vi "FollowerWall.vi"() -> ()   [LabVIEW 2016]
uses:
  <vilib>/NXT/Block Support/NXT_InputPort.ctl
  <vilib>/NXT/Block Support/NXT_TimerIndex.ctl
  <vilib>/NXT/Block Support/NXT_OutputPort.ctl
  <vilib>/NXT/Dual Mode Library/Sensors/EV3_Gyro_Reset.vi
  <vilib>/NXT/Dual Mode Library/Sensors/EV3_Gyro_Angle.vi
  <vilib>/NXT/Dual Mode Library/Sensors/EV3_Gyro_Rate.vi
  <vilib>/NXT/Dual Mode Library/Sensors/Reset_Timer.vi
  <vilib>/NXT/Dual Mode Library/Sensors/EV3_Color_Reflect.vi
  <vilib>/NXT/Dual Mode Library/Sensors/Read_Timer.vi
  <vilib>/NXT/Dual Mode Library/Sensors/EV3_Ultrasonic_CM.vi
  <vilib>/NXT/Dual Mode Library/Display/drawText_Right.vi
  <vilib>/NXT/Dual Mode Library/prims/inRangeAndCoerce/inRangeAndCoerce_float.vi
  <vilib>/NXT/NXTIO Xnodes/NXTIONodeSubVIs/NXTMoveMotors.vi
  <vilib>/NXT/Dual Mode Library/Display/drawNumber.vi
  <vilib>/NXT/Dual Mode Library/Display/drawNumber_float.vi
  <vilib>/NXT/Dual Mode Library/Motors/Rotation.vi
  <vilib>/NXT/Dual Mode Library/Motors/ResetMotor.vi
  <vilib>/NXT/Dual Mode Library/Display/drawText.vi
  <vilib>/NXT/NXTIO Xnodes/NXTIONodeSubVIs/NXTStopMotors.vi
  <vilib>/NXT/Subs/LVHSConnector.ctl
  <vilib>/NXT/NXTIO Xnodes/AddressXNode/NXTIOAddress.xnode
  <vilib>/NXT/NXTIO Xnodes/NXTIOXNode/NXTIO.xnode
  <vilib>/NXT/LegoClasses/BrickReference/BrickReference.lvclass
panel:
  out "Value (msec)":u32
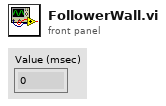
[diagram p1: front panel]
types:
  T1 = typedef "NXT_InputPort.ctl" = u32
  T2 = typedef "LVHSConnector.ctl" = refnum<class "BrickReference.lvclass">
  T3 = typedef "NXT_TimerIndex.ctl" = u8
  T4 = typedef "NXT_OutputPort.ctl" = u8
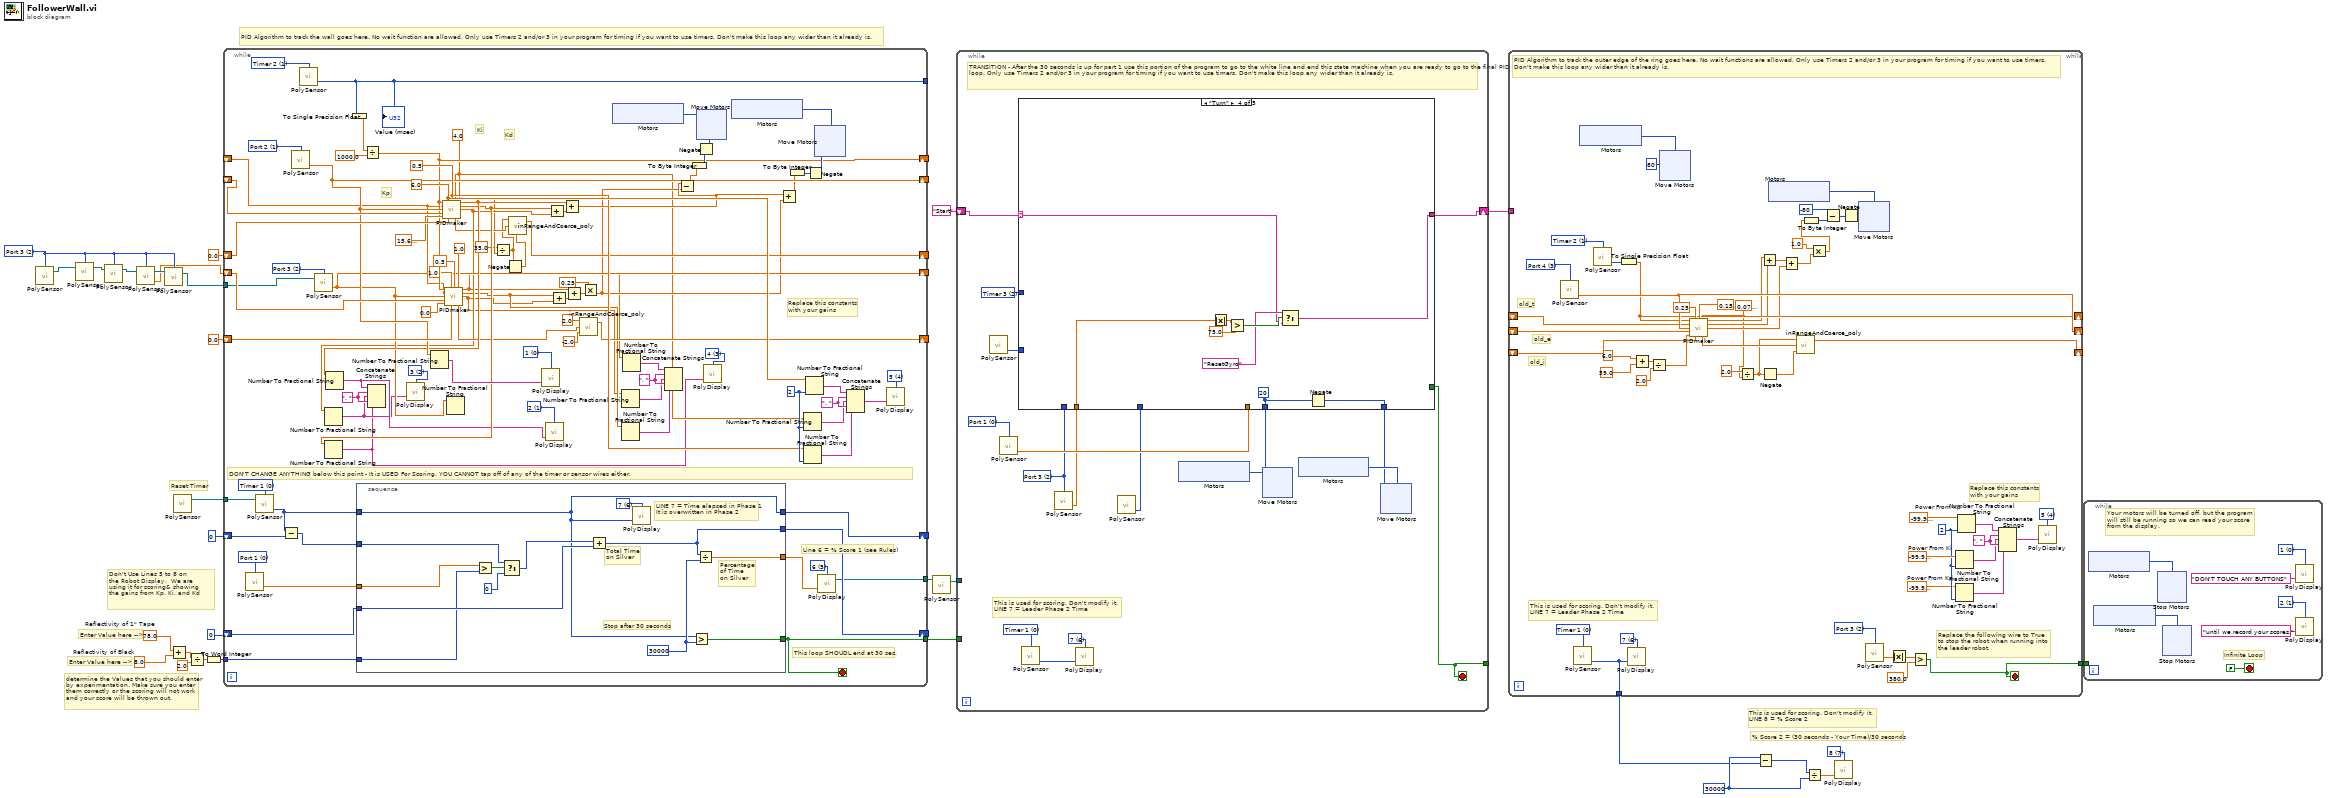
[diagram p0: block diagram]
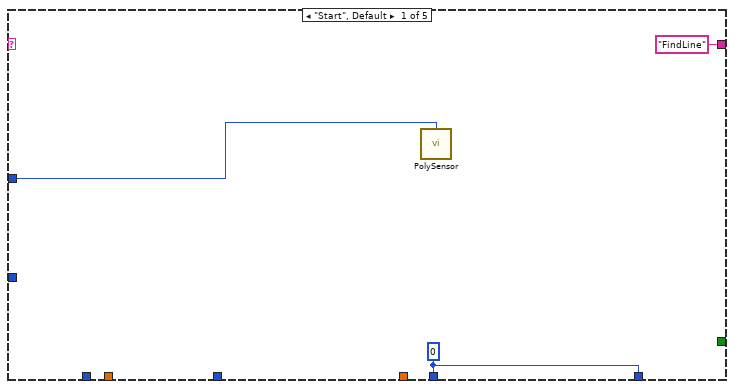
[diagram p2: hidden frame]
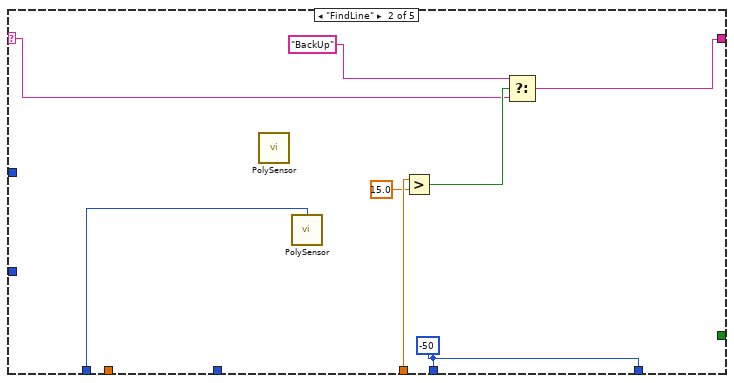
[diagram p3: hidden frame]
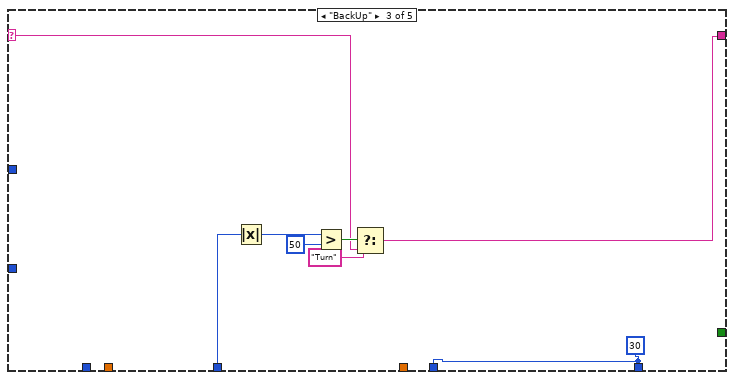
[diagram p4: hidden frame]
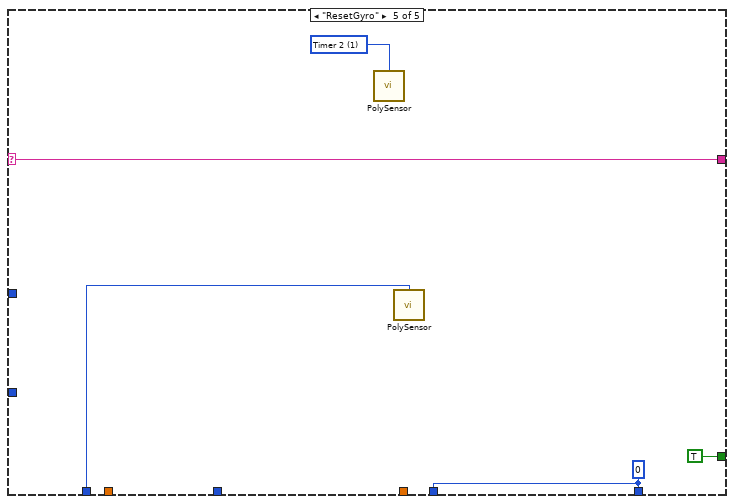
[diagram p5: hidden frame]
diagram:
  w5 = T1 2 items=["Port 1", "Port 2", "Port 3", "Port 4"] ("Port (Port 1)")
  w13 = u32 30000 ("Value (msec)")
  w14 = i16 7 items=["1", "2", "3", "4", "5", "6", "7", "8", "9", "10", "11", "12"] ("Line")
  w20 = 8.0  # Reflectivity of Black
  w19 = 78.0  # Reflectivity of 1" Tape
  # "PID Algorithm to track the wall goes here. No wait function are allowed. Only use Timers 2 and/or 3 in your program for timing if you want to use timers. Don't make this loop any wider than it already is."
  # "This is used for scoring. Don't modify it.\nLINE 8 = % Score 2"
  # "Don't Use Lines 5 to 8 on\nthe Robot Display.  We are \nusing it for scoring& showing \nthe gains from Kp, Ki, and Kd"
  # "% Score 2 = (30 seconds - Your Time)/30 seconds"
  # "Enter Value here -->"
  # "determine the Values that you should enter\nby experimentation. Make sure you enter \nthem correctly or the scoring will not work\nand your score will be thrown out."
  # "Enter Value here -->"
  # "Reset Timer"
  n1 = call-poly <vilib>:"PolySensor.vi"("Port (Port 1)"=w5) -> ("NXT/EV3"=w6:T2)  [unwired: 3 in]
  n2 = call-poly <vilib>:"PolySensor.vi"("NXT/EV3"=w6, "Port (Port 1)"=w5) -> ("NXT/EV3"=w7:T2)  [unwired: 1 in, 1 out]
  n3 = call-poly <vilib>:"PolySensor.vi"("NXT/EV3"=w7, "Port (Port 1)"=w5) -> ("NXT/EV3"=w9:T2)  [unwired: 1 in, 1 out]
  n4 = call-poly <vilib>:"PolySensor.vi"("NXT/EV3"=w9, "Port (Port 1)"=w5) -> ("Degrees"=w1:sgl, "NXT/EV3"=w8:T2)  [unwired: 1 in]
  n5 = call-poly <vilib>:"PolySensor.vi"("NXT/EV3"=w8, "Port (Port 1)"=w5) -> ("NXT/EV3"=w4:T2)  [unwired: 2 in]
  n6 = Add(x=w19, y=w20) -> (x+y=w18:dbl)
  n7 = call-poly <vilib>:"PolySensor.vi"() -> ("NXT/EV3"=w27:T2)  [unwired: 4 in]
  n8 = Divide(x=w18, y=2.0) -> (x/y=w17:dbl)
  n9 = To Word Integer(number=w17) -> (16bit integer=w24:i16)
  n10 = while {
    shift-right: [w113] -> _
    shift-left: i16 0 -> [w116]
    shift-right: [w114] -> _
    shift-left: i16 0 ("Value (msec)") -> [w115]
    tunnel: w27 -> [w112]
    tunnel: [w30] -> w26
    tunnel: w24 -> [w107]
    tunnel: [w103] -> w22
    shift-right: [w48] -> _
    shift-left: sgl 0.0 ("coerced(x)") -> [w84]
    shift-right: [w63] -> _
    shift-left: sgl 0.0 ("coerced(x)") -> [w89]
    shift-right: [w52] -> _
    shift-left: w1 -> [w87]
    tunnel: [w83] -> _
    shift-right: [w58] -> _
    shift-left: _ -> [w57]
    shift-right: [w71] -> _
    shift-left: _ -> [w79]
    tunnel: w4 -> [w51]
    stop <- w30 stop-if-true
    w44 = ", " ("string")
    w41 = i16 3 items=["1", "2", "3", "4", "5", "6", "7", "8", "9", "10", "11", "12"] ("Line")
    w53 = i16 1 items=["1", "2", "3", "4", "5", "6", "7", "8", "9", "10", "11", "12"] ("Line")
    w70 = ", " ("string")
    w69 = i16 2 items=["1", "2", "3", "4", "5", "6", "7", "8", "9", "10", "11", "12"] ("Line")
    w73 = i16 0 items=["1", "2", "3", "4", "5", "6", "7", "8", "9", "10", "11", "12"] ("Line")
    w37 = sgl 4.0 ("Ki")
    w76 = sgl 0.5 ("Kd")
    w77 = sgl 6.0 ("Kp")
    w80 = T1 1 items=["Port 1", "Port 2", "Port 3", "Port 4"] ("Port (Port 1)")
    w85 = T3 1 items=["Timer 1", "Timer 2", "Timer 3"] ("Timer (Timer 1)")
    w88 = T1 2 items=["Port 1", "Port 2", "Port 3", "Port 4"] ("Port (Port 1)")
    w99 = ", " ("string")
    w101 = i16 2 ("precision (6)")
    w102 = i16 4 items=["1", "2", "3", "4", "5", "6", "7", "8", "9", "10", "11", "12"] ("Line")
    w105 = i16 5 items=["1", "2", "3", "4", "5", "6", "7", "8", "9", "10", "11", "12"] ("Line")
    w109 = T1 0 items=["Port 1", "Port 2", "Port 3", "Port 4"] ("Port (Port 3)")
    w110 = T3 0 items=["Timer 1", "Timer 2", "Timer 3"] ("Timer (Timer 1)")
    # "Kp"
    # "Kd"
    # "Ki"
    # "Replace this constants\nwith your gains"
    # "DON'T CHANGE ANYTHING below this point - It is USED For Scoring. YOU CANNOT tap off of any of the timer or sensor wires either."
    # "Line 6 = % Score 1 (see Rules)"
    # "This loop SHOUDL end at 30 sec."
    n11 = call-poly <vilib>:"PolySensor.vi"("Port (Port 1)"=w109) -> ("Scaled Value"=w108:sgl)  [unwired: 2 in, 1 out]
    n12 = call-poly <vilib>:"PolySensor.vi"("NXT/EV3"=w112, "Timer (Timer 1)"=w110) -> ("Value (msec)"=w111:u32)  [unwired: 1 in, 1 out]
    n13 = Subtract(x=w111, y=w115) -> (x-y=w106:u32)
    n14 = call-poly <vilib>:"PolySensor.vi"("Port (Port 1)"=w80) -> ("Centimeters"=w71:sgl)  [unwired: 2 in, 1 out]
    n15 = call-poly <vilib>:"PolySensor.vi"("Timer (Timer 1)"=w85) -> ("Value (msec)"=w83:u32)  [unwired: 2 in, 1 out]
    "Value (msec)" <- w83
    n16 = call-poly <vilib>:"PolySensor.vi"("NXT/EV3"=w51, "Port (Port 1)"=w88) -> ("Degrees"=w52:sgl)  [unwired: 1 in, 1 out]
    n17 = To Single Precision Float(number=w83) -> (single precision float=w81:sgl)
    n18 = stacked-sequence {
      tunnel: w116 -> [w145]
      tunnel: [w135] -> w104
      tunnel: w111 -> [w133]
      tunnel: [w144] -> w30
      tunnel: w108 -> [w139]
      tunnel: w106 -> [w141]
      tunnel: [w133] -> w114
      tunnel: [w137] -> w113
      tunnel: w107 -> [w138]
      frame #0 {
        w134 = i16 6 items=["1", "2", "3", "4", "5", "6", "7", "8", "9", "10", "11", "12"] ("Line")
        w136 = u32 30000 ("Value (msec)")
        # "LINE 7 = Time elapsed in Phase 1\nIt is overwritten in Phase 2"
        # "Percentage\nof Time\non Silver"
        # "Stop after 30 seconds"
        # "Total Time\non Silver"
        n19 = Greater?(x=w139, y=w138) -> (0:w142:bool)
        n20 = Select(t=w141, s=w142, f=i16 0) -> (s? t:f=w140:u32)
        n21 = Add(x=w140, y=w145) -> (x+y=w137:u32)
        n22 = call-poly <vilib>:"PolyDisplay.vi"("number"=w133, "Line"=w134) -> ()  [unwired: 2 in, 1 out]
        n23 = Greater?(x=w133, y=w136) -> (0:w144:bool)
        n24 = Divide(x=w137, y=w136) -> (x/y=w135:dbl)
      }
    }
    n25 = Divide(x=w81, y=sgl 1000.0) -> (x/y=w58:sgl)
    n26 = Number To Fractional String(number=w71) -> (F-format string=w72:string)  [unwired: 3 in]
    n27 = call "PIDmaker.vi"("New Time"=w58, "Kp"=w77, "Kd"=w76, "Ki"=w37, "Old Time"=w57, "New Value"=w71, "Old Value"=w79, "Desired Value"=sgl 15.6, "Integral In"=w84) -> ("P out"=w68:sgl, "D out"=w67:sgl, "I out"=w50:sgl, "Integral Out"=w49:sgl)  [unwired: 3 in]
    n28 = Number To Fractional String(number=w50) -> (F-format string=w32:string)  [unwired: 3 in]
    n29 = Number To Fractional String(number=w67) -> (F-format string=w31:string)  [unwired: 3 in]
    n30 = Number To Fractional String(number=w68) -> (F-format string=w33:string)  [unwired: 3 in]
    n31 = Concatenate Strings(w33, w70, w32, w70, w31) -> ()  [unwired: 1 out]
    n32 = call-poly <vilib>:"PolyDisplay.vi"("Text"=w32, "Line"=w69) -> ()  [unwired: 2 in, 1 out]
    n33 = call "PIDmaker.vi"("New Time"=w58, "Kp"=sgl 1.0, "Kd"=sgl 0.5, "Ki"=sgl 1.0, "Old Time"=w57, "New Value"=w52, "Old Value"=w87, "Desired Value"=sgl 0.0, "Integral In"=w89) -> ("P out"=w40:sgl, "D out"=w39:sgl, "I out"=w38:sgl, "Integral Out"=w64:sgl)  [unwired: 3 in]
    n34 = Number To Fractional String(number=w52) -> ()  [unwired: 3 in, 1 out]
    n35 = Divide(x=sgl 35.0, y=w37) -> (x/y=w35:sgl)
    n36 = Negate(x=w35) -> (-x=w34:sgl)
    n37 = call-poly <vilib>:"inRangeAndCoerce_poly.vi"("lower limit"=w34, "x"=w49, "upper limit"=w35) -> ("coerced(x)"=w48:sgl)  [unwired: 1 out]
    n38 = call-poly <vilib>:"PolyDisplay.vi"("Text"=w72, "Line"=w73) -> ()  [unwired: 2 in, 1 out]
    n39 = call-poly <vilib>:"PolyDisplay.vi"("Text"=w33, "Line"=w53) -> ()  [unwired: 2 in, 1 out]
    n40 = Add(x=w67, y=w50) -> (x+y=w93:sgl)
    n41 = Add(x=w39, y=w38) -> (x+y=w90:sgl)
    n42 = Add(x=w68, y=w93) -> (x+y=w61:sgl)
    n43 = Add(x=w40, y=w90) -> (x+y=w59:sgl)
    n44 = call-poly <vilib>:"inRangeAndCoerce_poly.vi"("lower limit"=sgl -2.0, "x"=w64, "upper limit"=sgl 2.0) -> ("coerced(x)"=w63:sgl)  [unwired: 1 out]
    n45 = Multiply(x=sgl 0.25, y=w59) -> (x*y=w47:sgl)
    n46 = xnode "Motors"() -> ("Motor"=w95:T4)
    n47 = Number To Fractional String(number=w38) -> (F-format string=w43:string)  [unwired: 3 in]
    n48 = Number To Fractional String(number=w39) -> (F-format string=w42:string)  [unwired: 3 in]
    n49 = Number To Fractional String(number=w40) -> (F-format string=w45:string)  [unwired: 3 in]
    n50 = Concatenate Strings(w45, w44, w43, w44, w42) -> ()  [unwired: 1 out]
    n51 = Subtract(x=w61, y=w47) -> (x-y=w62:sgl)
    n52 = To Byte Integer(number=w62) -> (8bit integer=w74:i8)
    n53 = Negate(x=w74) -> (-x=w66:i8)
    n54 = xnode "Move Motors"("Power/Speed 1"=w66, "Motors"=w95) -> ()  [unwired: 1 in, 1 out]
    n55 = call-poly <vilib>:"PolyDisplay.vi"("Text"=w31, "Line"=w41) -> ()  [unwired: 2 in, 1 out]
    n56 = xnode "Motors"() -> ("Motor"=w94:T4)
    n57 = Add(x=w61, y=w47) -> (x+y=w60:sgl)
    n58 = To Byte Integer(number=w60) -> (8bit integer=w75:i8)
    n59 = Number To Fractional String(number=w37, precision (6)=w101) -> (F-format string=w98:string)  [unwired: 2 in]
    n60 = Number To Fractional String(number=w76, precision (6)=w101) -> (F-format string=w97:string)  [unwired: 2 in]
    n61 = Number To Fractional String(number=w77, precision (6)=w101) -> (F-format string=w100:string)  [unwired: 2 in]
    n62 = Negate(x=w75) -> (-x=w65:i8)
    n63 = xnode "Move Motors"("Power/Speed 1"=w65, "Motors"=w94) -> ()  [unwired: 1 in, 1 out]
    n64 = call-poly <vilib>:"PolyDisplay.vi"("number"=w104, "Line"=w105) -> ("NXT/EV3"=w103:T2)  [unwired: 2 in]
    n65 = Concatenate Strings(w100, w99, w98, w99, w97) -> (w96:string)
    n66 = call-poly <vilib>:"PolyDisplay.vi"("Text"=w96, "Line"=w102) -> ()  [unwired: 2 in, 1 out]
  }
  n67 = call-poly <vilib>:"PolySensor.vi"("NXT/EV3"=w22) -> ("NXT/EV3"=w21:T2)  [unwired: 3 in]
  n68 = while {
    tunnel: w26 -> [_]
    shift-right: [w149] -> w15
    shift-left: "Start" -> [w148]
    tunnel: w21 -> [_]
    tunnel: [w146] -> _
    stop <- w146 stop-if-true
    w147 = T1 0 items=["Port 1", "Port 2", "Port 3", "Port 4"] ("Port (Port 1)")
    w152 = T1 2 items=["Port 1", "Port 2", "Port 3", "Port 4"] ("Port (Port 1)")
    w157 = T3 2 items=["Timer 1", "Timer 2", "Timer 3"] ("Timer (Timer 1)")
    w160 = i16 6 items=["1", "2", "3", "4", "5", "6", "7", "8", "9", "10", "11", "12"] ("Line")
    w162 = T3 0 items=["Timer 1", "Timer 2", "Timer 3"] ("Timer (Timer 1)")
    # "This is used for scoring. Don't modify it.\nLINE 7 = Leader Phase 2 Time"
    # "TRANSITION - After the 30 seconds is up for part 1 use this portion of the program to go to the white line and end this state machine when you are ready to go to the final PID control loop. Only use Timers 2 and/or 3 in your program for timing if you want to use timers. Don't make this loop any wider than it already is."
    n69 = call-poly <vilib>:"PolySensor.vi"() -> ("Value (msec)"=w156:u32)  [unwired: 3 in, 1 out]
    n70 = call-poly <vilib>:"PolySensor.vi"("Port (Port 1)"=w147) -> ("Scaled Value"=w153:sgl)  [unwired: 2 in, 1 out]
    n71 = call-poly <vilib>:"PolySensor.vi"("Timer (Timer 1)"=w162) -> ("Value (msec)"=w161:u32)  [unwired: 2 in, 1 out]
    n72 = call-poly <vilib>:"PolySensor.vi"("Port (Port 1)"=w152) -> ("Degrees"=w151:sgl)  [unwired: 2 in, 1 out]
    n73 = call-poly <vilib>:"PolyDisplay.vi"("number"=w161, "Line"=w160) -> ()  [unwired: 2 in, 1 out]
    n74 = call-poly <vilib>:"PolySensor.vi"() -> ("Angle of Rotation"=w150:i32)  [unwired: 3 in, 1 out]
    n75 = case shown="\"Turn\"" w148 {
      selector: w148 -> [_ w184 w192 w199 w209]
      tunnel: ["FindLine" w186 w190 w198 w209] -> w149
      tunnel: w157 -> [w181 _ _ _ _]
      tunnel: w156 -> [_ _ _ _ _]
      tunnel: [w179 w182 w197 w206 w208] -> w155
      tunnel: [w179 w182 w197 w205 w208] -> w154
      tunnel: w153 -> [_ w189 _ _ _]
      tunnel: w152 -> [_ w183 _ _ w211]
      tunnel: w151 -> [_ _ _ w204 _]
      tunnel: w150 -> [_ _ w196 _ _]
      tunnel: [_ _ _ _ TRUE] -> w146
      frame "Start", Default {
        w179 = 0
        n76 = call-poly <vilib>:"PolySensor.vi"("Timer (Timer 1)"=w181) -> ()  [unwired: 3 in, 1 out]
      }
      frame "FindLine" {
        w182 = -50
        n77 = call-poly <vilib>:"PolySensor.vi"() -> ()  [unwired: 4 in, 1 out]
        n78 = call-poly <vilib>:"PolySensor.vi"("Port (Port 1)"=w183) -> ()  [unwired: 3 in, 1 out]
        n79 = Greater?(x=w189, y=sgl 15.0) -> (0:w187:bool)
        n80 = Select(t="BackUp", s=w187, f=w184) -> (s? t:f=w186:string)
      }
      frame "BackUp" {
        w197 = 30
        n81 = Absolute Value(x=w196) -> (abs(x)=w194:i32)
        n82 = Greater?(x=w194, y=50) -> (0:w193:bool)
        n83 = Select(t="Turn", s=w193, f=w192) -> (s? t:f=w190:string)
      }
      frame "Turn" {
        w206 = 20
        n84 = Absolute Value(x=w204) -> (abs(x)=w203:sgl)
        n85 = Greater?(x=w203, y=sgl 75.0) -> (0:w201:bool)
        n86 = Select(t="ResetGyro", s=w201, f=w199) -> (s? t:f=w198:string)
        n87 = Negate(x=w206) -> (-x=w205:i32)
      }
      frame "ResetGyro" {
        w207 = T3 1 items=["Timer 1", "Timer 2", "Timer 3"] ("Timer (Timer 1)")
        w208 = 0
        n88 = call-poly <vilib>:"PolySensor.vi"("Timer (Timer 1)"=w207) -> ()  [unwired: 3 in, 1 out]
        n89 = call-poly <vilib>:"PolySensor.vi"("Port (Port 1)"=w211) -> ()  [unwired: 3 in, 1 out]
      }
    }
    n90 = xnode "Motors"() -> ("Motor"=w159:T4)
    n91 = xnode "Move Motors"("Power/Speed 1"=w155, "Motors"=w159) -> ()  [unwired: 1 in, 1 out]
    n92 = xnode "Motors"() -> ("Motor"=w158:T4)
    n93 = xnode "Move Motors"("Power/Speed 1"=w154, "Motors"=w158) -> ()  [unwired: 1 in, 1 out]
  }
  n94 = while {
    tunnel: [w212] -> w16
    tunnel: w15 -> [_]
    tunnel: [w262] -> w12
    shift-right: [w247] -> _
    shift-left: _ -> [w246]
    shift-right: [w243] -> _
    shift-left: _ -> [w242]
    shift-right: [w230] -> _
    shift-left: _ -> [w231]
    stop <- w212 stop-if-true
    w216 = T1 2 items=["Port 1", "Port 2", "Port 3", "Port 4"] ("Port (Port 1)")
    w228 = sgl 0.07 ("Ki")
    w249 = T3 1 items=["Timer 1", "Timer 2", "Timer 3"] ("Timer (Timer 1)")
    w250 = T1 3 items=["Port 1", "Port 2", "Port 3", "Port 4"] ("Port (Port 1)")
    w255 = ", " ("string")
    w258 = i16 2 ("precision (6)")
    w257 = sgl -99.9  # Power From Kd
    w259 = sgl -99.9  # Power From Ki
    w260 = sgl -99.9  # Power From Kp
    w261 = i16 4 items=["1", "2", "3", "4", "5", "6", "7", "8", "9", "10", "11", "12"] ("Line")
    w263 = i16 6 items=["1", "2", "3", "4", "5", "6", "7", "8", "9", "10", "11", "12"] ("Line")
    w264 = T3 0 items=["Timer 1", "Timer 2", "Timer 3"] ("Timer (Timer 1)")
    # "old_i"
    # "old_e"
    # "old_t"
    # "Replace this constants\nwith your gains"
    # "This is used for scoring. Don't modify it.\nLINE 7 = Leader Phase 2 Time"
    # "PID Algorithm to track the outer edge of the ring goes here. No wait functions are allowed. Only use Timers 2 and/or 3 in your program for timing if you want to use timers.\nDon't make this loop any wider than it already is."
    # "Replace the following wire to True\nto stop the robot when running into \nthe leader robot."
    n95 = call-poly <vilib>:"PolySensor.vi"("Port (Port 1)"=w250) -> ("Scaled Value"=w247:sgl)  [unwired: 2 in, 1 out]
    n96 = call-poly <vilib>:"PolySensor.vi"("Timer (Timer 1)"=w264) -> ("Value (msec)"=w262:u32)  [unwired: 2 in, 1 out]
    n97 = xnode "Motors"() -> ("Motor"=w225:T4)
    n98 = call-poly <vilib>:"PolySensor.vi"("Timer (Timer 1)"=w249) -> ("Value (msec)"=w248:u32)  [unwired: 2 in, 1 out]
    n99 = To Single Precision Float(number=w248) -> (single precision float=w243:sgl)
    n100 = call-poly <vilib>:"PolyDisplay.vi"("number"=w262, "Line"=w263) -> ()  [unwired: 2 in, 1 out]
    n101 = Add(x=sgl 6.0, y=sgl 59.0) -> (x+y=w241:sgl)
    n102 = Divide(x=w241, y=sgl 2.0) -> (x/y=w238:sgl)
    n103 = xnode "Move Motors"("Power/Speed 1"=i8 80, "Motors"=w225) -> ()  [unwired: 1 in, 1 out]
    n104 = call "PIDmaker.vi"("New Time"=w243, "Kp"=sgl 0.25, "Kd"=sgl 0.15, "Ki"=w228, "Old Time"=w242, "New Value"=w247, "Old Value"=w246, "Desired Value"=w238, "Integral In"=w231) -> ("P out"=w234:sgl, "D out"=w233:sgl, "I out"=w232:sgl, "Integral Out"=w237:sgl)  [unwired: 3 in]
    n105 = Divide(x=sgl 2.0, y=w228) -> (x/y=w226:sgl)
    n106 = Add(x=w234, y=w233) -> (x+y=w235:sgl)
    n107 = Negate(x=w226) -> (-x=w227:sgl)
    n108 = xnode "Motors"() -> ("Motor"=w251:T4)
    n109 = Add(x=w235, y=w232) -> (x+y=w219:sgl)
    n110 = call-poly <vilib>:"inRangeAndCoerce_poly.vi"("lower limit"=w227, "x"=w237, "upper limit"=w226) -> ("coerced(x)"=w230:sgl)  [unwired: 1 out]
    n111 = Multiply(x=sgl 1.0 ("Ki"), y=w219) -> (x*y=w217:sgl)
    n112 = To Byte Integer(number=w217) -> (8bit integer=w223:i8)
    n113 = Subtract(x=i8 -80, y=w223) -> (x-y=w221:i8)
    n114 = Negate(x=w221) -> (-x=w220:i8)
    n115 = xnode "Move Motors"("Power/Speed 1"=w220, "Motors"=w251) -> ()  [unwired: 1 in, 1 out]
    n116 = call-poly <vilib>:"PolySensor.vi"("Port (Port 1)"=w216) -> ("Degrees"=w215:sgl)  [unwired: 2 in, 1 out]
    n117 = Absolute Value(x=w215) -> (abs(x)=w213:sgl)
    n118 = Greater?(x=w213, y=sgl 380.0) -> (0:w212:bool)
    n119 = Number To Fractional String(number=w259, precision (6)=w258) -> (F-format string=w254:string)  [unwired: 2 in]
    n120 = Number To Fractional String(number=w257, precision (6)=w258) -> (F-format string=w253:string)  [unwired: 2 in]
    n121 = Number To Fractional String(number=w260, precision (6)=w258) -> (F-format string=w256:string)  [unwired: 2 in]
    n122 = Concatenate Strings(w256, w255, w254, w255, w253) -> (w252:string)
    n123 = call-poly <vilib>:"PolyDisplay.vi"("Text"=w252, "Line"=w261) -> ()  [unwired: 2 in, 1 out]
  }
  n124 = Subtract(x=w13, y=w12) -> (x-y=w11:u32)
  n125 = Divide(x=w11, y=w13) -> (x/y=w10:dbl)
  n126 = call-poly <vilib>:"PolyDisplay.vi"("number"=w10, "Line"=w14) -> ()  [unwired: 2 in, 1 out]
  n127 = while {
    tunnel: w16 -> [_]
    stop <- FALSE stop-if-true
    w281 = i16 1 items=["1", "2", "3", "4", "5", "6", "7", "8", "9", "10", "11", "12"] ("Line")
    w284 = i16 0 items=["1", "2", "3", "4", "5", "6", "7", "8", "9", "10", "11", "12"] ("Line")
    # "Your motors will be turned off, but the program\nwill still be running so we can read your score\nfrom the display."
    # "Infinite Loop"
    n128 = xnode "Motors"() -> ("Motor"=w286:T4)
    n129 = xnode "Motors"() -> ("Motor"=w285:T4)
    n130 = xnode "Stop Motors"("Motors"=w286) -> ()  [unwired: 1 in, 1 out]
    n131 = xnode "Stop Motors"("Motors"=w285) -> ()  [unwired: 1 in, 1 out]
    n132 = call-poly <vilib>:"PolyDisplay.vi"("Text"="DON'T TOUCH ANY BUTTONS", "Line"=w284) -> ()  [unwired: 2 in, 1 out]
    n133 = call-poly <vilib>:"PolyDisplay.vi"("Text"="until we record your scores.", "Line"=w281) -> ()  [unwired: 2 in, 1 out]
  }
